vi "Run_clientSuper.vi"(11 "Path":path) -> (0 "error out":errorcluster, 3 "vi reference":refnum<vi>)   [LabVIEW 2019]
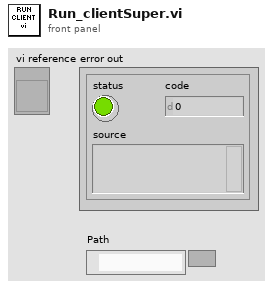
[diagram p1: front panel]
types:
  T1 = enum32{"Bad", "Idle", "Run top level", "Running"}
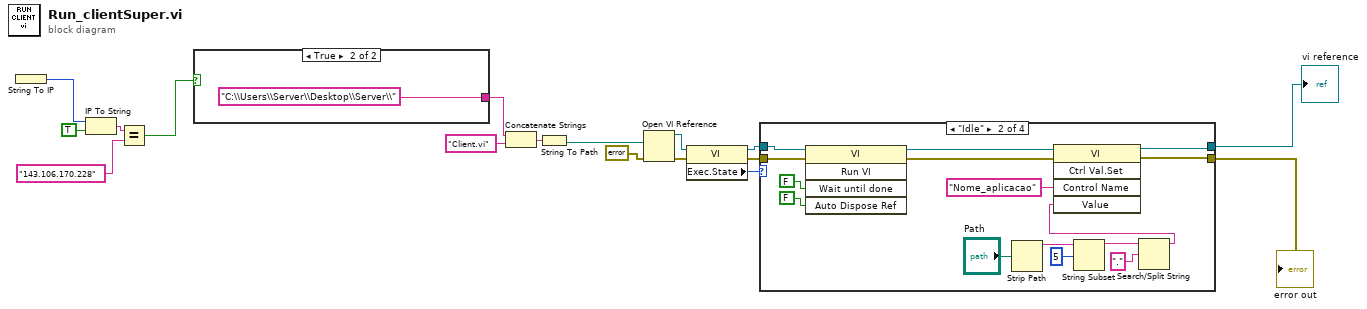
[diagram p0: block diagram]
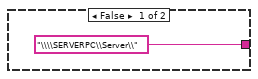
[diagram p2: hidden frame]
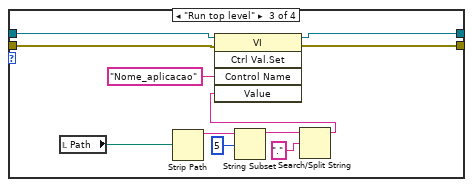
[diagram p4: hidden frame]
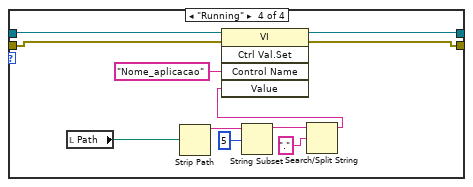
[diagram p5: hidden frame]
diagram:
  n1 = String To IP() -> (0:w5:u32)  [unwired: 1 in]
  n2 = IP To String(1:TRUE ("dot notation? (F)"), 2:w5) -> (0:w3:string)
  n3 = Equal?(x=w3, y="143.106.170.228" ("name")) -> (x = y?=w1:bool)
  n4 = case shown="True" w1 {
    tunnel: ["\\\\SERVERPC\\Server\\" "C:\\Users\\Server\\Desktop\\Server\\"] -> w10
    frame False {
    }
    frame True {
    }
  }
  n5 = Concatenate Strings(w10, "Client.vi" ("string")) -> (w9:string)
  n6 = String To Path(string=w9) -> (path=w16:path)
  n7 = Open VI Reference(vi path=w16, error in (no error)=errorcluster {"status"=FALSE, "code"=0, "source"=""}) -> (vi reference=w15:refnum<vi>, error out=w14:errorcluster)  [unwired: 4 in]
  n8 = property class="VI"(reference=w15, error in=w14) -> (reference out=w12:refnum<vi>, error out=w11:errorcluster, "Exec.State"=w13:T1)
  n9 = case shown="\"Idle\"" w13 {
    tunnel: [w21 w23 w40 w51] -> w7
    tunnel: [w20 w22 w39 w50] -> w6
    tunnel: w12 -> [w21 w34 w38 w49]
    tunnel: w11 -> [w20 w33 w37 w48]
    frame "Bad", Default {
    }
    frame "Idle" {
      n10 = invoke class="VI" method="Run VI"(reference=w34, error in=w33, "Wait until done"=FALSE ("Wait Until Done"), "Auto Dispose Ref"=FALSE ("Auto Dispose Reference")) -> (reference out=w25:refnum<vi>, error out=w24:errorcluster)  [unwired: 1 in, 3 out]
      n11 = Strip Path(path="Path") -> (name=w31:string)  [unwired: 1 out]
      n12 = String Subset(string=w31, offset (0)=5) -> (substring=w30:string)  [unwired: 1 in]
      n13 = Search/Split String(string=w30, search string/char (-)=".") -> (substring before match=w29:string)  [unwired: 1 in, 2 out]
      n14 = invoke class="VI" method="Ctrl Val.Set"(reference=w25, error in=w24, "Control Name"="Nome_aplicacao", "Value"=w29) -> (reference out=w23:refnum<vi>, error out=w22:errorcluster)  [unwired: 1 in, 3 out]
    }
    frame "Run top level" {
      n15 = local read "Path"() -> (w47:path)
      n16 = Strip Path(path=w47) -> (name=w46:string)  [unwired: 1 out]
      n17 = String Subset(string=w46, offset (0)=5) -> (substring=w45:string)  [unwired: 1 in]
      n18 = Search/Split String(string=w45, search string/char (-)=".") -> (substring before match=w44:string)  [unwired: 1 in, 2 out]
      n19 = invoke class="VI" method="Ctrl Val.Set"(reference=w38, error in=w37, "Control Name"="Nome_aplicacao", "Value"=w44) -> (reference out=w40:refnum<vi>, error out=w39:errorcluster)  [unwired: 1 in, 3 out]
    }
    frame "Running" {
      n20 = local read "Path"() -> (w58:path)
      n21 = Strip Path(path=w58) -> (name=w57:string)  [unwired: 1 out]
      n22 = String Subset(string=w57, offset (0)=5) -> (substring=w56:string)  [unwired: 1 in]
      n23 = Search/Split String(string=w56, search string/char (-)=".") -> (substring before match=w55:string)  [unwired: 1 in, 2 out]
      n24 = invoke class="VI" method="Ctrl Val.Set"(reference=w49, error in=w48, "Control Name"="Nome_aplicacao", "Value"=w55) -> (reference out=w51:refnum<vi>, error out=w50:errorcluster)  [unwired: 1 in, 3 out]
    }
  }
  "vi reference" <- w7
  "error out" <- w6
